vi "Error Converter (ErrCode or Status).vi"(8 "error in (no error)":errorcluster, 11 "error code":i32) -> (0 "error out":errorcluster)   [LabVIEW 2020, in "reqwest-labview.lvlib"]
uses:
  reqwest-labview.lvlib
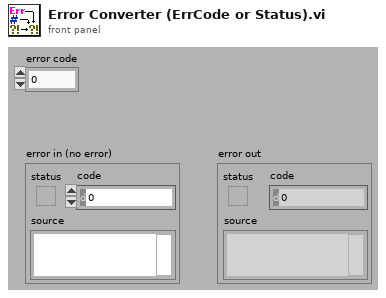
[diagram p1: front panel]
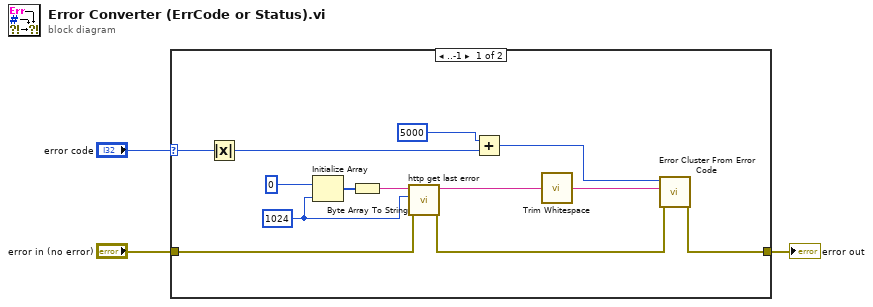
[diagram p0: block diagram]
diagram:
  n1 = case shown="..-1" "error code" {
    selector: "error code" -> [w8 _]
    tunnel: "error in (no error)" -> [w12 w17]
    tunnel: [w4 w17] -> w1
    frame ..-1 {
      w13 = 1024 ("dimension size")
      n2 = Absolute Value(x=w8) -> (abs(x)=w7:i32)
      n3 = Initialize Array(u8 0 ("unsigned 8bit integer"), w13) -> (w15:u8[])
      n4 = Byte Array To String(unsigned byte array=w15) -> (string=w14:string)
      n5 = call "http get last error.vi"("error in (no error)"=w12, "buf_len"=w13, "buf_ptr"=w14) -> ("error out"=w5:errorcluster, "buf_ptr out"=w11:string)  [unwired: 6 in, 1 out]
      n6 = Add(x=5000 ("error code (0)"), y=w7) -> (x+y=w6:i32)
      n7 = call <vilib>:"Trim Whitespace.vi"("string"=w11) -> ("trimmed string"=w10:string)  [unwired: 1 in]
      n8 = call <vilib>:"Error Cluster From Error Code.vi"("error in (no error)"=w5, "error message (\"\")"=w10, "error code (0)"=w6) -> ("error out"=w4:errorcluster)  [unwired: 6 in]
    }
    frame 0.. {
    }
  }
  "error out" <- w1
